vi "Anritsu VNA Read Format.vi"(6 "Channel":i8=1 min=1 max=99 step=1, 7 "Anritsu VNA":T1, 8 "error in (no error)":errorcluster, 11 "VISA Resource Name":refnum<visa-resource-name>) -> (0 "error out":errorcluster, 2 "Display Format":T2, 3 "dup VISA Resource Name":refnum<visa-resource-name>)   [LabVIEW 2011]
doc: "This VI for the HP 8753B is used to read the meausurement format.\n\n0 log magnitude\n1 phase\n2 delay\n3 Smith chart\n4 polar\n5 linear magnitude\n6 standing wave ratio\n7 real\n8 imaginary"
uses:
  tests/S Parameter/TypeDefs/SP Measurement Format.ctl
  TypeDefs/Anritsu VNA Instrument Info.ctl
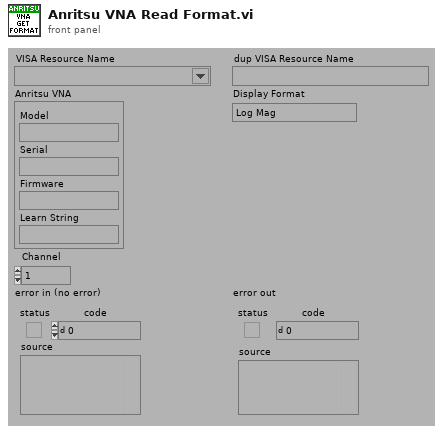
[diagram p1: front panel]
types:
  T1 = typedef "Anritsu VNA Instrument Info.ctl" = cluster{"Model":string, "Serial":string, "Firmware":string, "Learn String":string}
  T2 = typedef "SP Measurement Format.ctl" = enum32{"Log Mag", "Phase", "Delay", "Smith (R+jX)", "Polar (Re/Im)", "Linear Mag", "SWR", "Real", "Imaginary", "Smith (Lin/Phase)", "Smith (Log/Phase)", "Smith (Real/Imag)", "Smith (G+jB)", "Polar (Lin/Phase)", "Polar (Log/Phase)", "Expanded Phase", "Positive Phase", "Inverted Smith", "Unwrapped Phase", "Power Out", "Power In", "Linear Mag/Phase", "Log Mag/Phase", "Real/Imaginary"}
  T3 = typedef "Anritsu VNA Model.ctl" = enum16{"Not Supported", "37XXXX", "MS20XXX", "MS462XX", "MS464XX"}
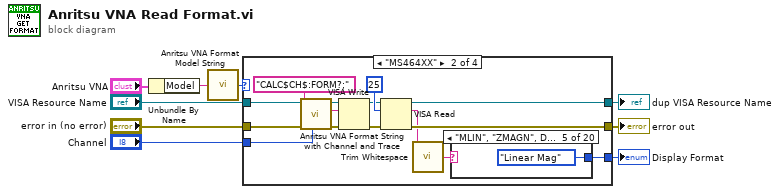
[diagram p0: block diagram]
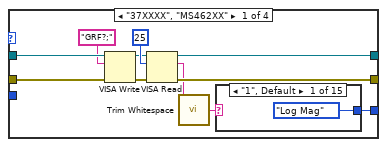
[diagram p2: hidden frame]
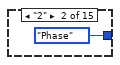
[diagram p3: hidden frame]
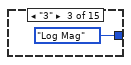
[diagram p4: hidden frame]
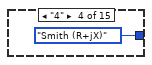
[diagram p5: hidden frame]
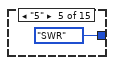
[diagram p6: hidden frame]
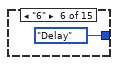
[diagram p7: hidden frame]
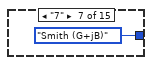
[diagram p8: hidden frame]
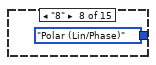
[diagram p9: hidden frame]
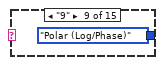
[diagram p10: hidden frame]
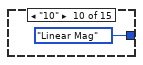
[diagram p11: hidden frame]
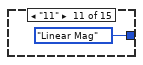
[diagram p12: hidden frame]
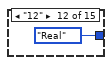
[diagram p13: hidden frame]
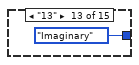
[diagram p14: hidden frame]
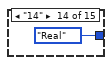
[diagram p15: hidden frame]
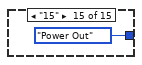
[diagram p16: hidden frame]
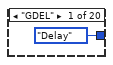
[diagram p17: hidden frame]
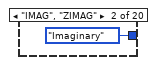
[diagram p18: hidden frame]
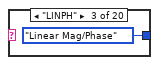
[diagram p19: hidden frame]
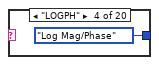
[diagram p20: hidden frame]
diagram:
  n1 = Unbundle By Name("Anritsu VNA") -> ("Model"=w3:string)
  n2 = call "Anritsu VNA Format Model String.vi"("Model"=w3) -> ("Model"=w2:T3)
  n3 = case shown="\"MS464XX\"" w2 {
    tunnel: "error in (no error)" -> [w14 w42 w71 w74]
    tunnel: [w17 w45 w71 w74] -> w8
    tunnel: [w11 w39 SP_Measurement_Format."Log Mag" ("Display Format") SP_Measurement_Format."Real" ("Display Format")] -> w7
    tunnel: "VISA Resource Name" -> [w15 w43 w70 w73]
    tunnel: [w16 w44 w70 w73] -> w5
    tunnel: "Channel" -> [_ w36 _ _]
    frame "37XXXX", "MS462XX" {
      n4 = VISA Write(VISA resource name=w15, write buffer="GRF?;", error in (no error)=w14) -> (VISA resource name out=w19:refnum<visa-resource-name>, error out=w18:errorcluster)  [unwired: 1 out]
      n5 = VISA Read(VISA resource name=w19, byte count=u32 25, error in (no error)=w18) -> (VISA resource name out=w16:refnum<visa-resource-name>, read buffer=w13:string, error out=w17:errorcluster)  [unwired: 1 out]
      n6 = call <vilib>:"Trim Whitespace.vi"("string"=w13) -> ("trimmed string"=w12:string)  [unwired: 1 in]
      n7 = case shown="\"1\", Default" w12 {
        tunnel: [SP_Measurement_Format."Log Mag" ("Display Format") SP_Measurement_Format."Phase" ("Display Format") SP_Measurement_Format."Log Mag" ("Display Format") SP_Measurement_Format."Smith (R+jX)" ("Display Format") SP_Measurement_Format."SWR" ("Display Format") SP_Measurement_Format."Delay" ("Display Format") SP_Measurement_Format."Smith (G+jB)" ("Display Format") SP_Measurement_Format."Polar (Lin/Phase)" ("Display Format") SP_Measurement_Format."Polar (Log/Phase)" ("Display Format") SP_Measurement_Format."Linear Mag" ("Display Format") SP_Measurement_Format."Linear Mag" ("Display Format") SP_Measurement_Format."Real" ("Display Format") SP_Measurement_Format."Imaginary" ("Display Format") SP_Measurement_Format."Real" ("Display Format") SP_Measurement_Format."Power Out" ("Display Format")] -> w11
        frame "1", Default {
        }
        frame "2" {
        }
        frame "3" {
        }
        frame "4" {
        }
        frame "5" {
        }
        frame "6" {
        }
        frame "7" {
        }
        frame "8" {
        }
        frame "9" {
        }
        frame "10" {
        }
        frame "11" {
        }
        frame "12" {
        }
        frame "13" {
        }
        frame "14" {
        }
        frame "15" {
        }
      }
    }
    frame "MS464XX" {
      n8 = call "Anritsu VNA Format String with Channel and Trace.vi"("Channel"=w36, "String"="CALC$CH$:FORM?;") -> ("String Out"=w38:string)  [unwired: 1 in, 6 out]
      n9 = VISA Write(VISA resource name=w43, write buffer=w38, error in (no error)=w42) -> (VISA resource name out=w47:refnum<visa-resource-name>, error out=w46:errorcluster)  [unwired: 1 out]
      n10 = VISA Read(VISA resource name=w47, byte count=u32 25, error in (no error)=w46) -> (VISA resource name out=w44:refnum<visa-resource-name>, read buffer=w41:string, error out=w45:errorcluster)  [unwired: 1 out]
      n11 = call <vilib>:"Trim Whitespace.vi"("string"=w41) -> ("trimmed string"=w40:string)  [unwired: 1 in]
      n12 = case shown="\"MLIN\", \"ZMAGN\", Default" w40 {
        tunnel: [SP_Measurement_Format."Delay" ("Display Format") SP_Measurement_Format."Imaginary" ("Display Format") SP_Measurement_Format."Linear Mag/Phase" ("Display Format") SP_Measurement_Format."Log Mag/Phase" ("Display Format") SP_Measurement_Format."Linear Mag" ("Display Format") SP_Measurement_Format."Log Mag" ("Display Format") SP_Measurement_Format."Phase" ("Display Format") SP_Measurement_Format."Polar (Lin/Phase)" ("Display Format") SP_Measurement_Format."Polar (Log/Phase)" ("Display Format") SP_Measurement_Format."Polar (Re/Im)" ("Display Format") SP_Measurement_Format."Power In" ("Display Format") SP_Measurement_Format."Power Out" ("Display Format") SP_Measurement_Format."Real" ("Display Format") SP_Measurement_Format."Real/Imaginary" ("Display Format") SP_Measurement_Format."Smith (Real/Imag)" ("Display Format") SP_Measurement_Format."Smith (Lin/Phase)" ("Display Format") SP_Measurement_Format."Smith (Log/Phase)" ("Display Format") SP_Measurement_Format."Smith (G+jB)" ("Display Format") SP_Measurement_Format."Smith (R+jX)" ("Display Format") SP_Measurement_Format."SWR" ("Display Format")] -> w39
        frame "GDEL" {
        }
        frame "IMAG", "ZIMAG" {
        }
        frame "LINPH" {
        }
        frame "LOGPH" {
        }
        frame "MLIN", "ZMAGN", Default {
        }
        frame "MLOG" {
        }
        frame "PHAS" {
        }
        frame "PLIN" {
        }
        frame "PLOG" {
        }
        frame "PLINCOMP", "PLOGCOMP" {
        }
        frame "PWRI" {
        }
        frame "PWRO" {
        }
        frame "REAL", "ZREAL" {
        }
        frame "REIM", "ZCOMP" {
        }
        frame "SADCOMP", "SCOMP" {
        }
        frame "SADLIN", "SLIN" {
        }
        frame "SADLOG", "SLOG" {
        }
        frame "SADM" {
        }
        frame "SMIT" {
        }
        frame "SWR" {
        }
      }
    }
    frame "Not Supported" {
    }
    frame "MS20XXX" {
    }
  }
  "Display Format" <- w7
  "dup VISA Resource Name" <- w5
  "error out" <- w8
